vi "1.vi"() -> ()   [LabVIEW 2015]
panel:
  in  "Stop":bool
  in  "Start":bool
  in  "Delta":i32(slide) scale=0.0..500.0
  out "Temperature":T1(graph)
  in  "High Limit":dbl
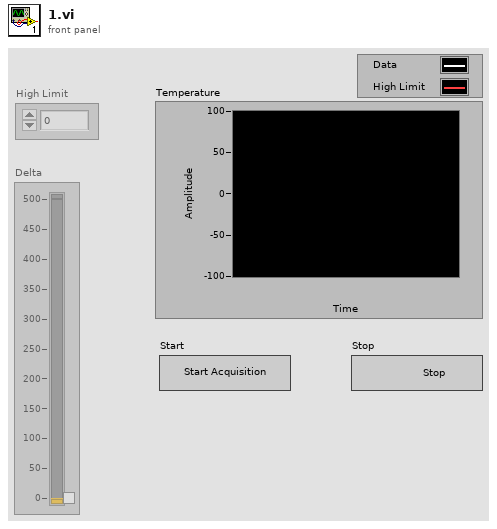
[diagram p1: front panel]
types:
  T1 = cluster{"Temperature Value":dbl, "Numeric Control":dbl}
  T2 = cluster{"Temperature Value":dbl, "Numeric Control":dbl}[]
  T3 = enum8{"Enabled", "Disabled", "Disabled and Grayed Out"}
  T4 = cluster{"Temperature Value":dbl, "High Limit":dbl}
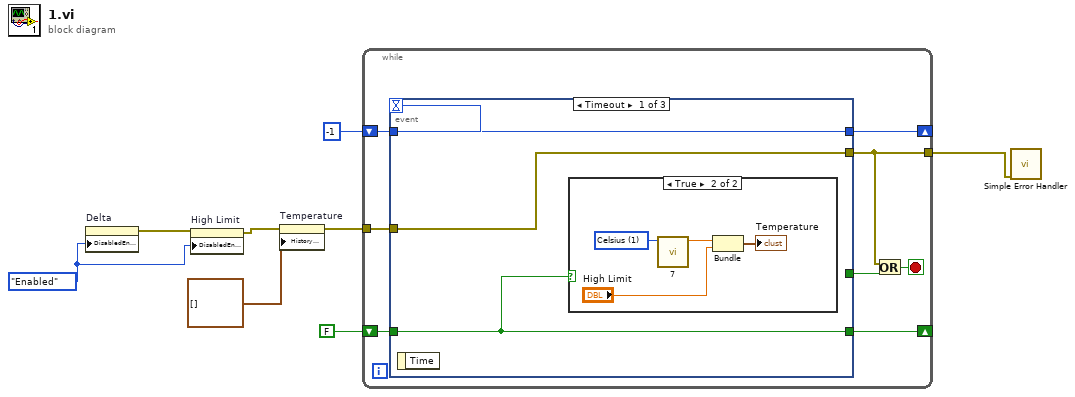
[diagram p0: block diagram]
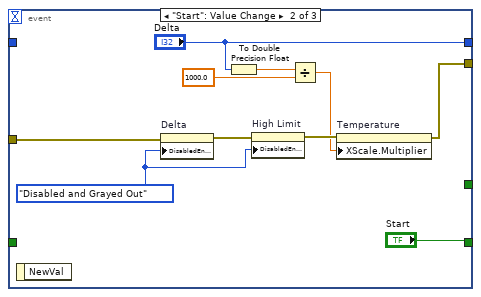
[diagram p3: hidden frame]
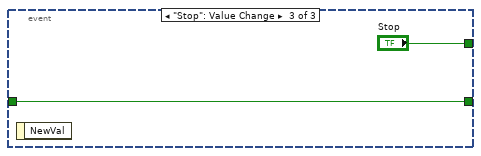
[diagram p4: hidden frame]
diagram:
  w4 = T3."Enabled" ("Disabled")
  n1 = property on="Delta" class="Slide (strict)"("DisabledEnum"=w4) -> (error out=w5:errorcluster)  [unwired: 2 in, 1 out]
  n2 = property on="High Limit" class="DigNum (strict)"(error in=w5, "DisabledEnum"=w4) -> (error out=w6:errorcluster)  [unwired: 1 in, 1 out]
  n3 = property on="Temperature" class="WFChart (strict)"(error in=w6, "History Data"=T2 []) -> (error out=w2:errorcluster)  [unwired: 1 in, 1 out]
  n4 = while {
    shift-right: [w16] -> _
    shift-left: -1 -> [w15]
    shift-right: [w13] -> _
    shift-left: FALSE -> [w14]
    tunnel: w2 -> [w11]
    tunnel: [w10] -> w1
    stop <- w12 stop-if-true
    n5 = event shown="[0] Timeout" {
      selector: _ -> [_ _ _]
      dyn-events: _ -> [_ _ _]
      timeout: w15 -> [_ _ _]
      tunnel: w15 -> [w19 _ _]
      tunnel: [w19 "Delta" _] -> w16
      tunnel: w14 -> [w18 _ w34]
      tunnel: [w18 "Start" w34] -> w13
      tunnel: w11 -> [w17 w30 _]
      tunnel: [w17 w26 _] -> w10
      tunnel: [_ _ "Stop"] -> w9
      event Timeout {
        n6 = event-data() -> ()  [unwired: 1 in, 1 out]
        n7 = case shown="True" w18 {
          frame False {
          }
          frame True {
            w23 = u16 1 items=["Fahrenheit", "Celsius"] ("Unit (0: Celsius)")
            n8 = call "7.vi"("Unit (0: Celsius)"=w23) -> ("Temperature Value"=w22:dbl)  [unwired: 10 in]
            n9 = Bundle("Temperature Value"=w22, "High Limit"="High Limit") -> (→"Temperature":T4)  [unwired: 1 in]
          }
        }
      }
      event "Start": Value Change {
        w28 = T3."Disabled and Grayed Out" ("Disabled")
        n10 = event-data() -> ()  [unwired: 1 in, 1 out]
        n11 = property on="Delta" class="Slide (strict)"(error in=w30, "DisabledEnum"=w28) -> (error out=w29:errorcluster)  [unwired: 1 in, 1 out]
        n12 = To Double Precision Float(number="Delta") -> (double precision float=w33:dbl)
        n13 = property on="High Limit" class="DigNum (strict)"(error in=w29, "DisabledEnum"=w28) -> (error out=w27:errorcluster)  [unwired: 1 in, 1 out]
        n14 = Divide(x=w33, y=1000.0) -> (x/y=w24:dbl)
        n15 = property on="Temperature" class="WFChart (strict)"(error in=w27, "XScale.Multiplier"=w24) -> (error out=w26:errorcluster)  [unwired: 1 in, 1 out]
      }
      event "Stop": Value Change {
        n16 = event-data() -> ()  [unwired: 1 in, 1 out]
      }
    }
    n17 = Or(x=w10, y=w9) -> (x .or. y?=w12:bool)
  }
  n18 = call <vilib>:"Simple Error Handler.vi"("error in (no error)"=w1) -> ()  [unwired: 4 in, 5 out]
